vi "Measurement UI.vi"() -> ()   [LabVIEW 2021, in "Single Tone_Audio DAC_UI.lvlib"]
uses:
  Single Tone_Audio DAC_UI.lvlib
  shared/audio popup ui/Audio Popup UI.lvlib
  Single Tone_Audio DAC.lvlib
panel:
  out "Frequency domain graph":cluster{"x0":dbl, "dx":dbl, "magnitude":dbl[]}[](graph)
  out "Time domain graph":waveform(dbl)[](graph)
  out "Table results":string[][](table)
  in  "settings tab":T1(tab)
  in  "Min settling time (s)":dbl=0.1 caption="MINIMUM SETTLING TIME" format="%#_6ps"
  in  "Min settling cycles":u32 caption="MINIMUM SETTLING CYCLES"
  in  "Min measurement time (s)":dbl=0.1 caption="MINIMUM MEASUREMENT TIME" format="%#_6ps"
  in  "Min measurement cycles":u32 caption="MINIMUM MEASUREMENT CYCLES"
  in  "Sample rate (Hz)":dbl=51200.0 caption="SAMPLE RATE" format="%#_6pHz"
  in  "Acquisition channel":string caption="ACQUISITION CHANNEL"
  in  "Output range (Vpk-pk)":dbl=5.74 caption="OUTPUT RANGE" format="%.3p Vpk-pk"
  in  "Output level units":string(combo)="dBFS"
  in  "Output level":dbl=-1.0 caption="OUTPUT LEVEL" format="%#_6p"
  in  "Frequency (Hz)":dbl=1000.0 caption="FREQUENCY" format="%#_6pHz"
  in  "Master clock channel":string caption="MASTER CLOCK CHANNEL"
  in  "Digital audio channel":string caption="DIGITAL AUDIO CHANNEL"
  out "digital serial file name":string
  in  "configure digital serial":bool
  in  "Gain units":string(combo)="dB" caption="Gain"
  in  "THD units":string(combo)="dB" caption="THD"
  in  "THD+N units":string(combo)="dB" caption="THD + N"
  in  "SNR units":string(combo)="dB" caption="SNR"
  in  "Band stop (Hz)":dbl=20000.0 caption="BAND STOP" format="%#_6pHz"
  in  "Band start (Hz)":dbl=20.0 caption="BAND START" format="%#_6pHz"
  in  "Weighting filter":string(combo)="A-weighting" caption="WEIGHTING FILTER"
  in  "Lowpass filter":string(combo)="No filter" caption="LOWPASS FILTER"
  in  "Highpass filter":string(combo)="AC" caption="HIGHPASS FILTER"
  out "Gain":dbl[](array[numeric]) format="%_6g"
  out "THD":dbl[](array[numeric]) format="%_6g"
  out "THD+N":dbl[](array[numeric]) format="%_6g"
  out "SNR":dbl[](array[numeric]) format="%_6g"
  out "SFDR (dBc)":dbl[](array[numeric]) format="%_6g"
  out "Dynamic range (dB)":dbl[](array[numeric]) format="%_6g"
  out "Phase (deg)":dbl[](array[numeric]) format="%_6g"
  out "Amplitude (dB)":dbl[](array[numeric]) format="%_6g"
  out "Amplitude (V)":dbl[](array[numeric]) format="%_6g"
  out "Frequency (Hz)":dbl[](array[numeric]) format="%_6g"
  out "df":dbl format="%_6g"
  out "f0":dbl format="%_6g"
  out "dt":dbl format="%_6g"
  out "Frequency domain":dbl[](array[numeric]) format="%_6g"
  out "Time domain":dbl[](array[numeric]) format="%_6g"
  out "Channel names":string[](array[string])
  in  "Protocol file":string
  # "Protocol settings"
  # "Generation settings"
  # "Acquisition settings"
  # "Filters"
  # "Units"
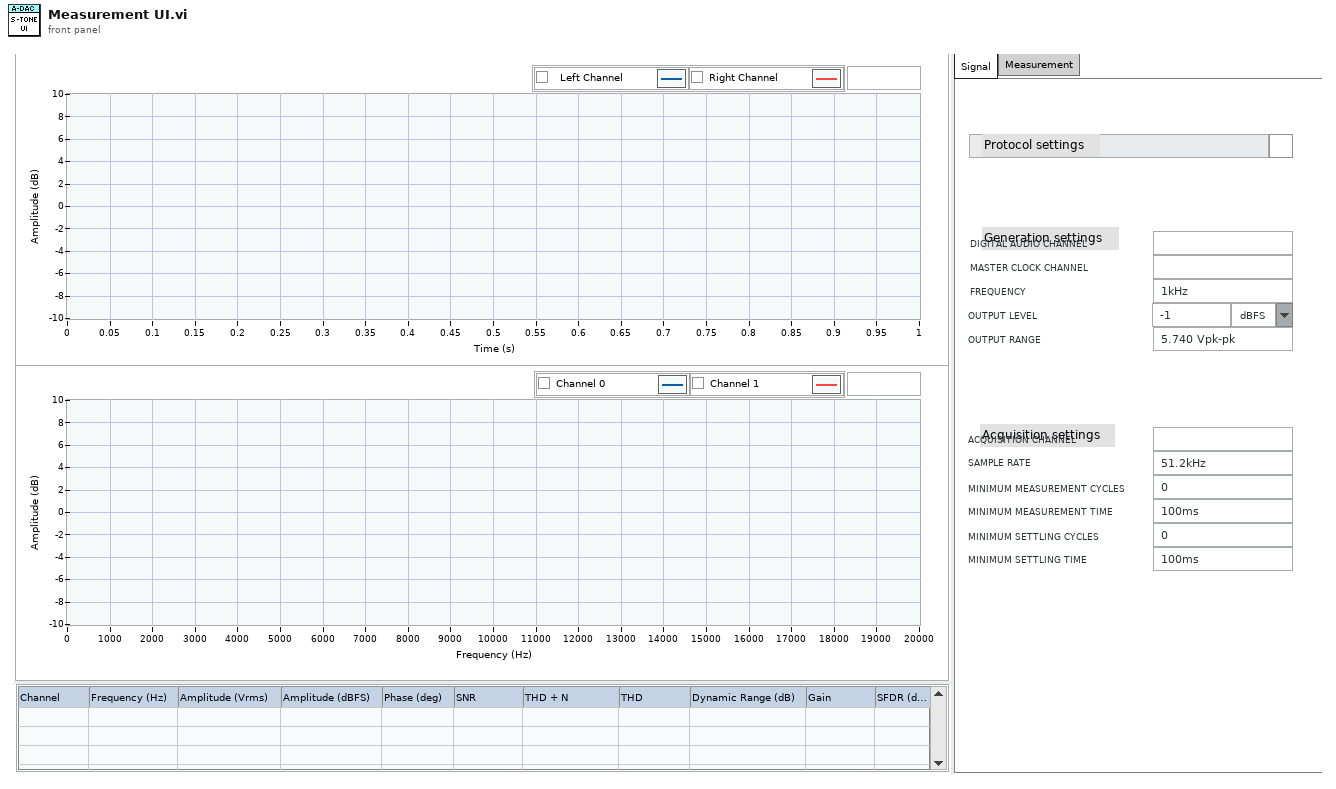
[diagram p1: front panel]
types:
  T1 = enum32{"Signal", "Measurement", "HiddenControls"}
  T2 = cluster{"Channel names":refnum<vi>, "Frequency (Hz)":refnum<vi>, "Amplitude (V)":refnum<vi>, "Amplitude (dB)":refnum<vi>, "Phase (deg)":refnum<vi>, "SNR":refnum<vi>, "THD+N":refnum<vi>, "THD":refnum<vi>, "Dynamic range (dB)":refnum<vi>, "Gain":refnum<vi>, "SFDR (dBc)":refnum<vi>, "SNR units":refnum<vi>, "THD+N units":refnum<vi>, "THD units":refnum<vi>, "Gain units":refnum<vi>}
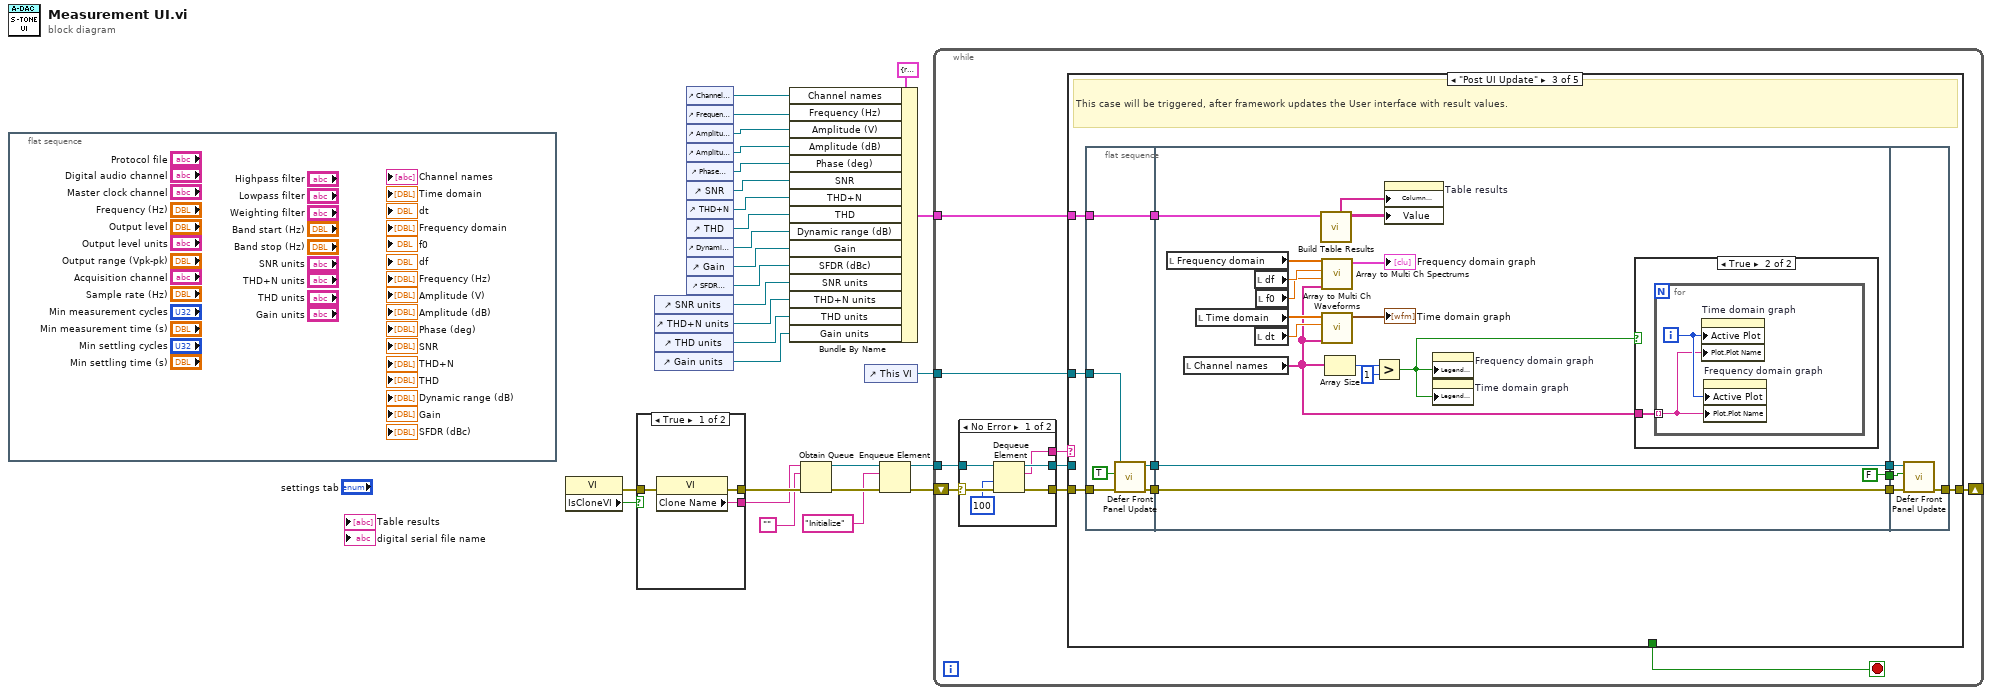
[diagram p0: block diagram]
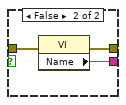
[diagram p2: hidden frame]
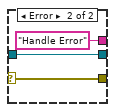
[diagram p3: hidden frame]
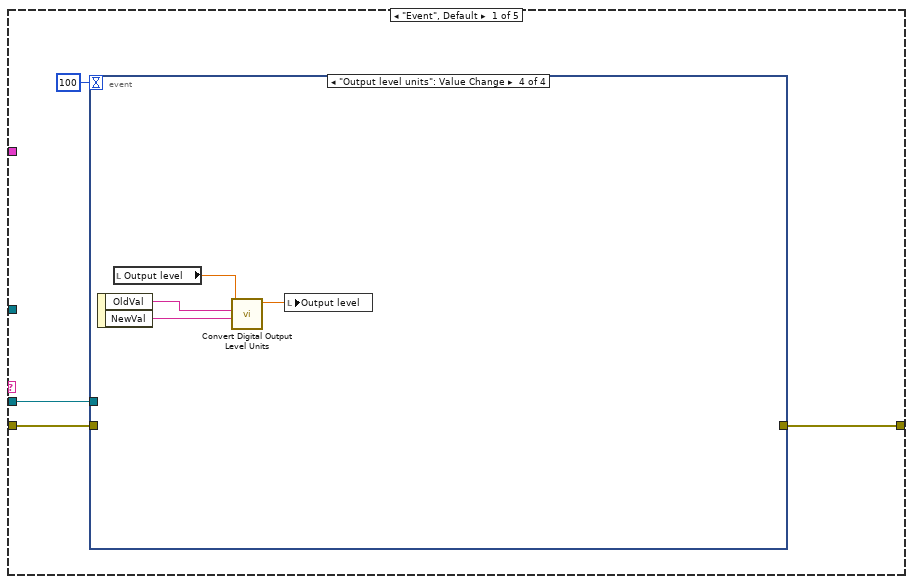
[diagram p4: hidden frame]
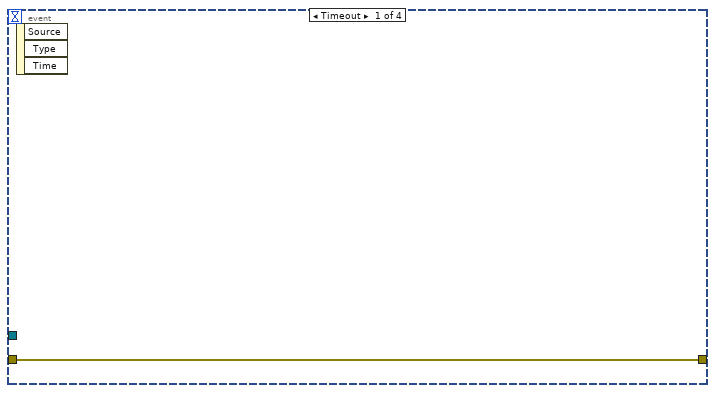
[diagram p5: hidden frame]
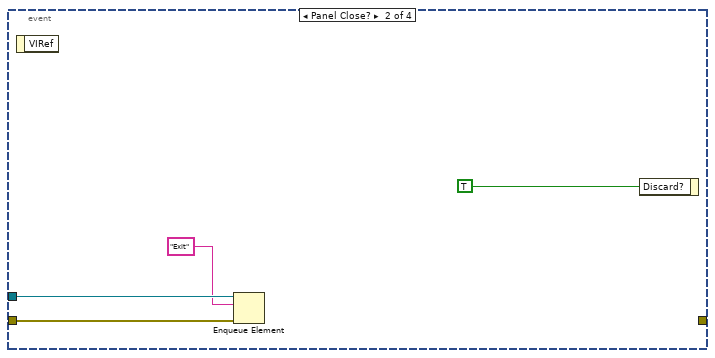
[diagram p6: hidden frame]
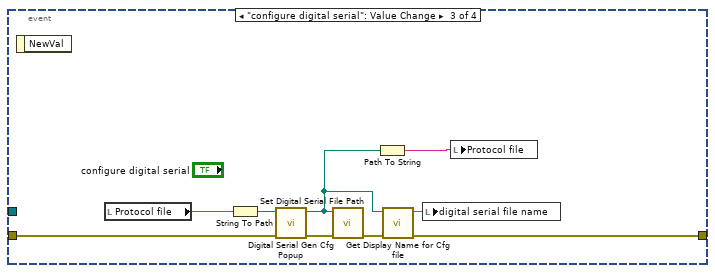
[diagram p7: hidden frame]
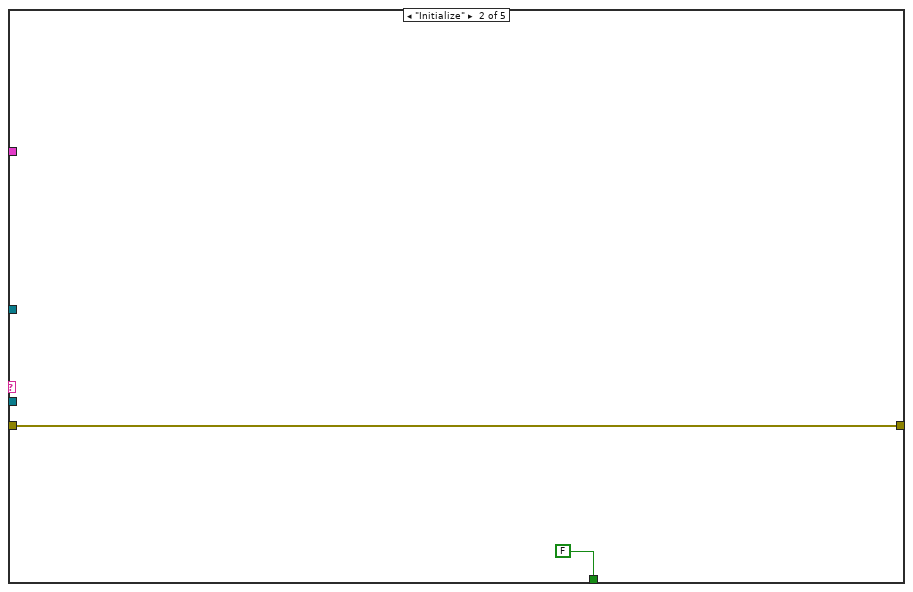
[diagram p8: hidden frame]
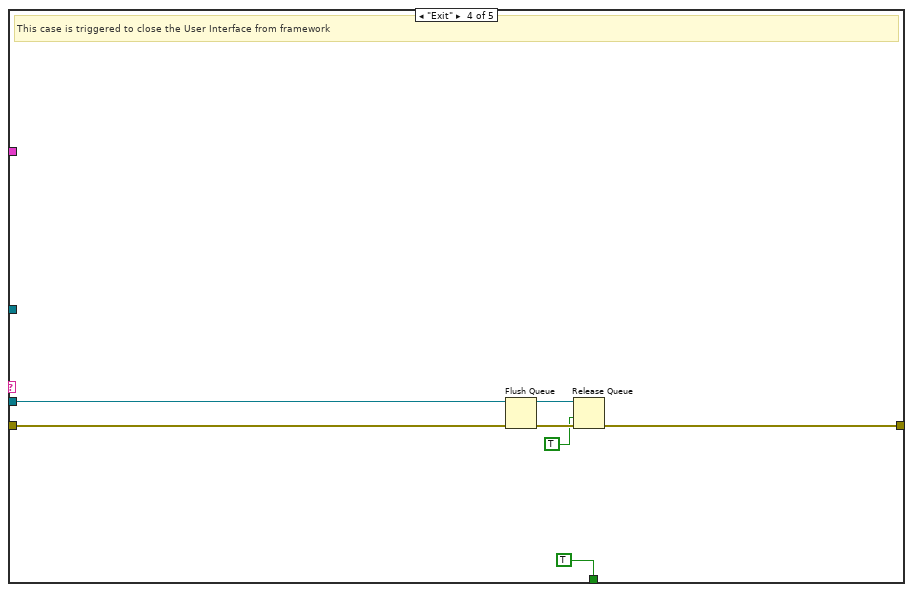
[diagram p10: hidden frame]
diagram:
  n1 = flat-sequence {
    frame #0 {
    }
  }
  n2 = property class="VI"() -> (error out=w19:errorcluster, "IsCloneVI"=w20:bool)  [unwired: 2 in, 1 out]
  n3 = case shown="True" w20 {
    tunnel: [w31 w34] -> w28
    tunnel: [w30 w33] -> w27
    tunnel: w19 -> [w29 w32]
    frame True {
      n4 = property class="VI"(error in=w29) -> (error out=w31:errorcluster, "Clone Name"=w30:string)  [unwired: 1 in, 1 out]
    }
    frame False {
      n5 = property class="VI"(error in=w32) -> (error out=w34:errorcluster, "Name"=w33:string)  [unwired: 1 in, 1 out]
    }
  }
  n6 = control-ref of="SNR units"() -> (w15:refnum<vi>)
  n7 = control-ref of="THD+N units"() -> (w16:refnum<vi>)
  n8 = control-ref of="THD units"() -> (w17:refnum<vi>)
  n9 = control-ref of="Gain units"() -> (w18:refnum<vi>)
  n10 = control-ref of="Channel names"() -> (w4:refnum<vi>)
  n11 = control-ref of="Frequency (Hz)"() -> (w5:refnum<vi>)
  n12 = control-ref of="Amplitude (V)"() -> (w6:refnum<vi>)
  n13 = control-ref of="Amplitude (dB)"() -> (w7:refnum<vi>)
  n14 = control-ref of="Phase (deg)"() -> (w8:refnum<vi>)
  n15 = control-ref of="SNR"() -> (w9:refnum<vi>)
  n16 = control-ref of="THD+N"() -> (w10:refnum<vi>)
  n17 = control-ref of="THD"() -> (w11:refnum<vi>)
  n18 = control-ref of="Dynamic range (dB)"() -> (w12:refnum<vi>)
  n19 = control-ref of="Gain"() -> (w13:refnum<vi>)
  n20 = control-ref of="SFDR (dBc)"() -> (w14:refnum<vi>)
  n21 = Bundle By Name(cluster=T2 {"Channel names"=refnum, "Frequency (Hz)"=refnum, "Amplitude (V)"=refnum, "Amplitude (dB)"=refnum, "Phase (deg)"=refnum, "SNR"=refnum, "THD+N"=refnum, "THD"=refnum, "Dynamic range (dB)"=refnum, "Gain"=refnum, "SFDR (dBc)"=refnum, "SNR units"=refnum, "THD+N units"=refnum, "THD units"=refnum, "Gain units"=refnum} ("output cluster"), "Channel names"=w4, "Frequency (Hz)"=w5, "Amplitude (V)"=w6, "Amplitude (dB)"=w7, "Phase (deg)"=w8, "SNR"=w9, "THD+N"=w10, "THD"=w11, "Dynamic range (dB)"=w12, "Gain"=w13, "SFDR (dBc)"=w14, "SNR units"=w15, "THD+N units"=w16, "THD units"=w17, "Gain units"=w18) -> (w2:T2)
  n22 = Obtain Queue(name (unnamed)=w27, element data type="", error in (no error)=w28) -> (queue out=w24:refnum<queue>, error out=w26:errorcluster)  [unwired: 2 in, 1 out]
  n23 = control-ref of="This VI"() -> (w1:refnum<vi>)
  n24 = Enqueue Element(queue=w24, element="Initialize", error in (no error)=w26) -> (queue out=w23:refnum<queue>, error out=w25:errorcluster)  [unwired: 1 in, 1 out]
  n25 = while {
    shift-right: [w38] -> _
    shift-left: w25 -> [w43]
    tunnel: w23 -> [w41]
    tunnel: w2 -> [w36]
    tunnel: w1 -> [w35]
    stop <- w37 stop-if-true
    n26 = case shown="No Error" w43 {
      selector: w43 -> [w49 w52]
      tunnel: [w48 w52] -> w42
      tunnel: w41 -> [w47 w51]
      tunnel: [w46 w51] -> w40
      tunnel: [w45 "Handle Error"] -> w39
      frame No Error {
        n27 = Dequeue Element(queue=w47, timeout in ms (-1)=100, error in (no error)=w49) -> (queue out=w46:refnum<queue>, element=w45:string, error out=w48:errorcluster)  [unwired: 1 out]
      }
      frame Error {
      }
    }
    n28 = case shown="\"Post UI Update\"" w39 {
      tunnel: w42 -> [w55 w76 w83 w123 w124]
      tunnel: w40 -> [w53 _ _ w121 _]
      tunnel: [w56 w76 w80 w118 w124] -> w38
      tunnel: [_ FALSE _ TRUE _] -> w37
      tunnel: w36 -> [_ _ w86 _ _]
      tunnel: w35 -> [_ _ w84 _ _]
      frame "Event", Default {
        n29 = event shown="[3] \"Output level units\": Value Change" {
          selector: _ -> [_ _ _ _]
          dyn-events: _ -> [_ _ _ _]
          timeout: 100 -> [_ _ _ _]
          tunnel: [w57 _ w67 _] -> w56
          tunnel: w55 -> [w57 w60 w70 _]
          tunnel: w53 -> [_ w59 _ _]
          event Timeout {
            n30 = event-data() -> ()  [unwired: 1 in, 3 out]
          }
          event Panel Close? {
            n31 = event-data() -> ()  [unwired: 1 in, 1 out]
            n32 = Enqueue Element(queue=w59, element="Exit", error in (no error)=w60) -> ()  [unwired: 1 in, 3 out]
            n33 = event-data("Discard?"=TRUE) -> ()  [unwired: 1 in, 1 out]
          }
          event "configure digital serial": Value Change {
            n34 = event-data() -> ()  [unwired: 1 in, 1 out]
            n35 = local read "Protocol file"() -> (w65:string)
            n36 = String To Path(string=w65) -> (path=w64:path)
            n37 = call "Digital Serial Gen Cfg Popup.vi"("error in (no error)"=w70, "config file in"=w64) -> ("error out"=w69:errorcluster, "config file out"=w63:path)  [unwired: 7 in, 1 out]
            n38 = call "Set Digital Serial File Path.vi"("error in (no error)"=w69, "digital serial file"=w63) -> ("error out"=w68:errorcluster)  [unwired: 9 in]
            n39 = Path To String(path=w63) -> (string=w62:string)
            n40 = call "Get Display Name for Cfg file.vi"("error in (no error)"=w68, "file path"=w63) -> ("error out"=w67:errorcluster, "display string"=w66:string)  [unwired: 8 in]
            n41 = local write "digital serial file name"(w66) -> ()
            n42 = local write "Protocol file"(w62) -> ()
          }
          event "Output level units": Value Change {
            n43 = event-data() -> ("OldVal"=w74:string, "NewVal"=w73:string)  [unwired: 1 in]
            n44 = local read "Output level"() -> (w72:dbl)
            n45 = call "Convert Digital Output Level Units.vi"("New output level units"=w73, "Previous output level units"=w74, "Previous output level"=w72) -> ("New output level"=w71:dbl)  [unwired: 8 in]
            n46 = local write "Output level"(w71) -> ()
          }
        }
      }
      frame "Initialize" {
      }
      frame "Post UI Update" {
        # "This case will be triggered, after framework updates the User interface with result values."
        n47 = flat-sequence {
          tunnel: w86 -> [w92]
          tunnel: [w92] -> w85
          tunnel: w84 -> [w90]
          tunnel: w83 -> [w89]
          tunnel: [w88] -> w81
          tunnel: [w87] -> w79
          tunnel: w85 -> [w100]
          tunnel: [w95] -> w82
          tunnel: w81 -> [w95]
          tunnel: w79 -> [w94]
          tunnel: [w94] -> w78
          tunnel: [FALSE] -> w77
          tunnel: w82 -> [w116]
          tunnel: [w115] -> w80
          tunnel: w78 -> [w114]
          tunnel: w77 -> [w113]
          frame #0 {
            n48 = call "Defer Front Panel Update.vi"("error in (no error)"=w89, "Defer Panel Updates"=TRUE, "VI in"=w90) -> ("error out"=w88:errorcluster, "VI out"=w87:refnum<vi>)  [unwired: 7 in]
          }
          frame #1 {
            n49 = local read "Frequency domain"() -> (w106:dbl[])
            n50 = local read "Channel names"() -> (w96:string[])
            n51 = local read "Time domain"() -> (w108:dbl[])
            n52 = local read "df"() -> (w105:dbl)
            n53 = local read "dt"() -> (w107:dbl)
            n54 = local read "f0"() -> (w104:dbl)
            n55 = call "Build Table Results.vi"("Table result references"=w100) -> ("Table values"=w98:string[][], "Column headers"=w99:string[])  [unwired: 9 in]
            n56 = call "Array to Multi Ch Spectrums.vi"("channel names"=w96, "f0"=w104, "df"=w105, "array"=w106) -> ("spectra"=→"Frequency domain graph":cluster{"x0":dbl, "dx":dbl, "magnitude":dbl[]}[])  [unwired: 7 in]
            n57 = call "Array to Multi Ch Waveforms.vi"("channel names"=w96, "dt"=w107, "array"=w108) -> ("waveforms"=→"Time domain graph":waveform(dbl)[])  [unwired: 8 in]
            n58 = Array Size(array=w96) -> (size(s)=w102:i32)
            n59 = Greater?(x=w102, y=1) -> (0:w97:bool)
            n60 = property on="Table results" class="Tbl (strict)"("Column Headers[]"=w99, "Value"=w98) -> ()  [unwired: 2 in, 2 out]
            n61 = property on="Frequency domain graph" class="WFGraph (strict)"("Legend Visible"=w97) -> ()  [unwired: 2 in, 2 out]
            n62 = property on="Time domain graph" class="WFGraph (strict)"("Legend Visible"=w97) -> ()  [unwired: 2 in, 2 out]
            n63 = case shown="True" w97 {
              tunnel: w96 -> [_ w110]
              frame False {
              }
              frame True {
                n64 = for {
                  tunnel: w110 -> [w111] mode=indexing
                  i -> [w112]
                  n65 = property on="Time domain graph" class="WFGraph (strict)"("Active Plot"=w112, "Plot.Plot Name"=w111) -> ()  [unwired: 2 in, 2 out]
                  n66 = property on="Frequency domain graph" class="WFGraph (strict)"("Active Plot"=w112, "Plot.Plot Name"=w111) -> ()  [unwired: 2 in, 2 out]
                }
              }
            }
          }
          frame #2 {
            n67 = call "Defer Front Panel Update.vi"("error in (no error)"=w116, "Defer Panel Updates"=w113, "VI in"=w114) -> ("error out"=w115:errorcluster)  [unwired: 7 in, 1 out]
          }
        }
      }
      frame "Exit" {
        # "This case is triggered to close the User Interface from framework"
        n68 = Flush Queue(queue=w121, error in (no error)=w123) -> (queue out=w120:refnum<queue>, error out=w119:errorcluster)  [unwired: 1 out]
        n69 = Release Queue(queue=w120, force destroy? (F)=TRUE, error in (no error)=w119) -> (error out=w118:errorcluster)  [unwired: 2 out]
      }
      frame "Handle Error" {
      }
    }
  }
